vi "SpecificVI - Modal Calling VI.vi"(10 "Sequence Context In":refnum<k7>, 11 "Description":string) -> ()   [LabVIEW 2009]
panel:
  in  "stop":bool
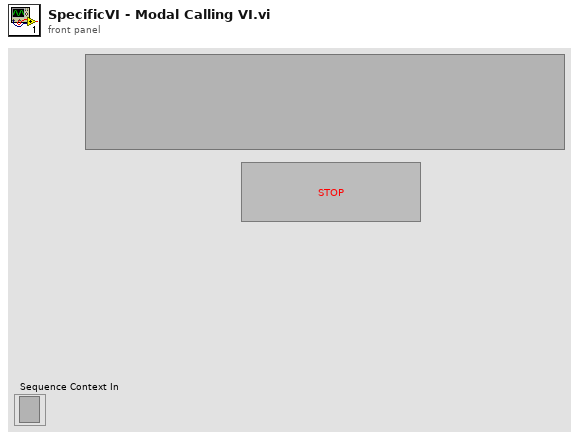
[diagram p1: front panel]
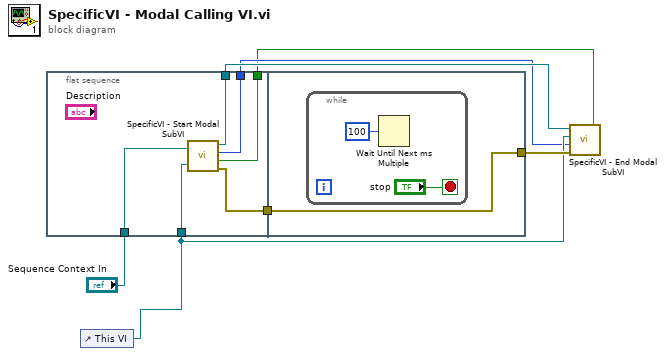
[diagram p0: block diagram]
diagram:
  n1 = flat-sequence {
    tunnel: w4 -> [w13]
    tunnel: [w12] -> w7
    tunnel: [w11] -> w5
    tunnel: [w10] -> w3
    tunnel: [w9] -> w2
    tunnel: "Sequence Context In" -> [w8]
    tunnel: w7 -> [w14]
    tunnel: [w14] -> w6
    frame #0 {
      n2 = call "SpecificVI - Start Modal SubVI.vi"("Sequence Context In"=w8, "This VI"=w13) -> ("Sequence Context Out"=w11:refnum<k7>, "Modal ID"=w10:i32, "VI Originally Open"=w9:bool, "error out"=w12:errorcluster)
    }
    frame #1 {
      n3 = while {
        stop <- "stop" stop-if-true
        n4 = Wait Until Next ms Multiple(millisecond multiple=u32 100) -> ()  [unwired: 1 out]
      }
    }
  }
  n5 = control-ref of="This VI"() -> (w4:refnum<vi>)
  n6 = call "SpecificVI - End Modal SubVI.vi"("VI Originally Open"=w2, "error out"=w6, "Modal ID"=w3, "This VI"=w4, "Sequence Context Out"=w5) -> ()
